vi "Custom Unflatten From String.vi"(9 "byte order (0:big-endian, network order)":T1(ring)=enum."little-endian", 10 "data includes array or string size? (T)":bool=TRUE, 11 "binary string":string="\u000f\u0000\u0000\u0000{\"source\":\"NT\"}\u0011\u0012E") -> (2 "value":string, 3 "rest of the binary string":string)   [LabVIEW 2023]
panel:
  out "Number of bytes in data":i32
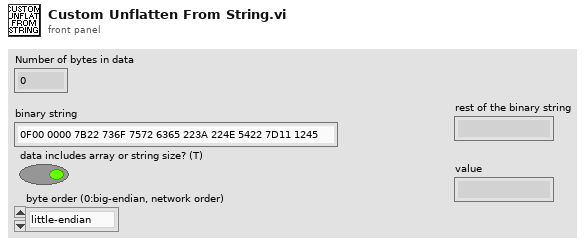
[diagram p1: front panel]
types:
  T1 = enum16{"big-endian, network order", "native, host order", "little-endian"}
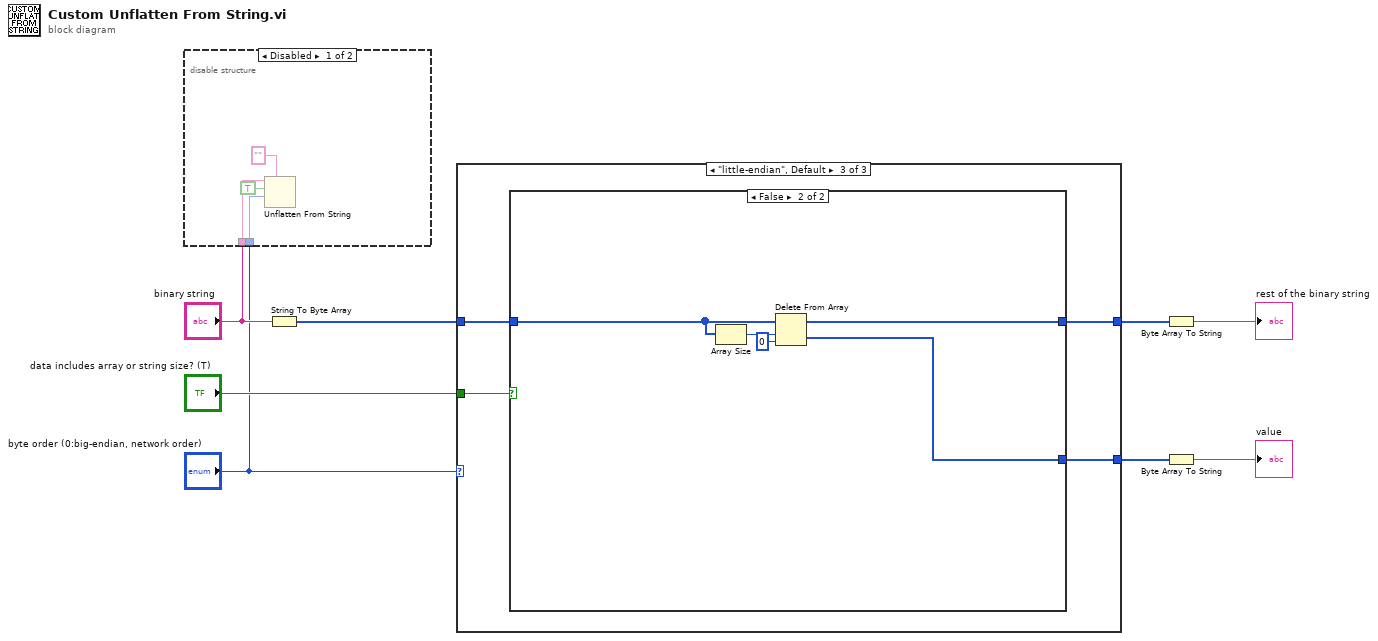
[diagram p0: block diagram]
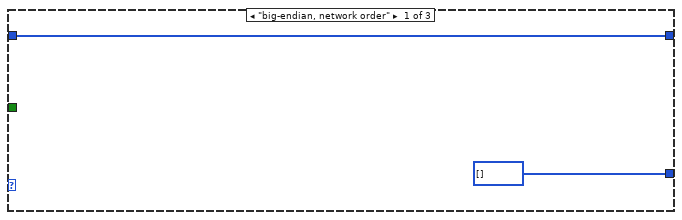
[diagram p3: hidden frame]
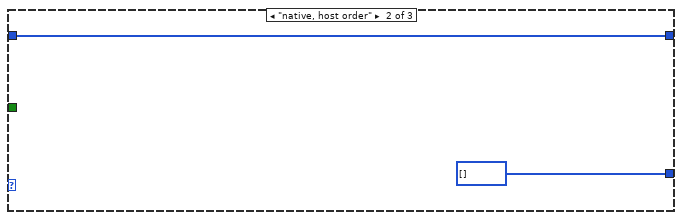
[diagram p4: hidden frame]
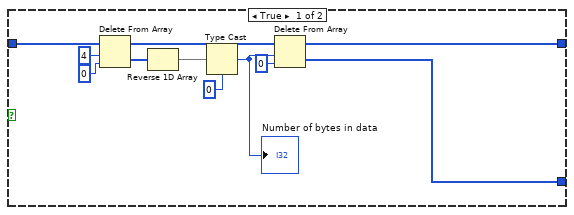
[diagram p5: hidden frame]
diagram:
  n1 = disable-structure shown="Disabled" {
    disable-tunnel: "binary string" -> [w12 _]
    disable-tunnel: "byte order (0:big-endian, network order)" -> [w10 _]
    frame Disabled {
      n2 = Unflatten From String(type="", binary string=w12, data includes array or string size? (T)=TRUE, byte order (0:big-endian, network order)=w10) -> ()  [unwired: 1 in, 3 out]
    }
    frame Enabled {
    }
  }
  n3 = String To Byte Array(string="binary string") -> (unsigned byte array=w7:u8[])
  n4 = case shown="\"little-endian\", Default" "byte order (0:big-endian, network order)" {
    tunnel: "data includes array or string size? (T)" -> [_ _ w19]
    tunnel: w7 -> [w14 w16 w20]
    tunnel: [w14 w16 w18] -> w3
    tunnel: [u8[] [] ("unsigned byte array") u8[] [] ("unsigned byte array") w17] -> w4
    frame "big-endian, network order" {
    }
    frame "native, host order" {
    }
    frame "little-endian", Default {
      n5 = case shown="False" w19 {
        tunnel: w20 -> [w31 w33]
        tunnel: [w22 w35] -> w18
        tunnel: [w21 w34] -> w17
        frame True {
          n6 = Delete From Array(array=w31, length=4, index=0) -> (deleted portion=w30:u8[], array with subset deleted=w25:u8[])
          n7 = Reverse 1D Array(array=w30) -> (reversed array=w29:u8[])
          n8 = Type Cast(type=0, x=w29) -> (*(type *) &x=w24:i32)
          "Number of bytes in data" <- w24
          n9 = Delete From Array(array=w25, length=w24, index=0) -> (deleted portion=w21:u8[], array with subset deleted=w22:u8[])
        }
        frame False {
          n10 = Array Size(array=w33) -> (size(s)=w32:i32)
          n11 = Delete From Array(array=w33, length=w32, index=0) -> (deleted portion=w34:u8[], array with subset deleted=w35:u8[])
        }
      }
    }
  }
  n12 = Byte Array To String(unsigned byte array=w3) -> (string=→"rest of the binary string":string)
  n13 = Byte Array To String(unsigned byte array=w4) -> (string=→"value":string)
